vi "Power Output Retrieve Key Array for  Config.vi"(8 "error in (no error)":errorcluster, 9 "Datasheets":T11, 10 "Key Array In":T12, 11 "Connection Refnum":T1) -> (0 "error out":errorcluster, 2 "Power Output Test Parameters":T2={"Stimulus"={"Frequency Type"=enum."Band Edges", "Frequency Ranges"=[], "TX 1 Frequency (MHz)"={"Min"=0.0, "Max"=0.0}, "TX 2 Frequency (MHz)"={"Min"=0.0, "Max"=0.0}, "RX Frequency (MHz)"={"Min"=0.0, "Max"=0.0}, "Pad Model Number"="", "Pad Serial Number"="", "Pad Values"=[]}, "Measurement"={"DUT Port"=enum."Port 1", "Direction"=0, "Frequency Step Size"=0}, "Display"={"Frequency"={"Min"=-1.0, "Max"=-1.0}, "Power"={"Min"=-1, "Max"=-1}}, "Limit"={"Min Power (dBm)"=44.0}, "Calibration"={"Calibrated?"=FALSE}} {"Measurement"."Frequency Step Size" items=["0.2", "0.4", "1.0", "2.0", "4.0"]; "Measurement"."Direction" items=["Reverse", "Forward", "Auxiliary"]}, 3 "Connection Refnum":T1)   [LabVIEW 2011]
uses:
  Addons/internet/utils/keyedarr.llb/Keyed Array.ctl
  Test Datasheets.ctl
  TypeDefs/Power Output Test Parameters.ctl
  TypeDefs/Power Output Stimulus Parameters.ctl
  TypeDefs/Power Output Measurement Parameters.ctl
  SI.LIB/PIM.LIB/HW IO/DUTport.ctl
  SI.LIB/PIM.LIB/HW IO/MeasMode.ctl
  SI.LIB/PIM.LIB/HW IO/PIM Sweep Step Size.ctl
  TypeDefs/Power Output Display Parameters.ctl
  TypeDefs/Power Output Limit Parameters.ctl
  TypeDefs/Power Output Calibration State.ctl
  SI.LIB/ODBC/SQL Controls/Connection Refnum.ctl
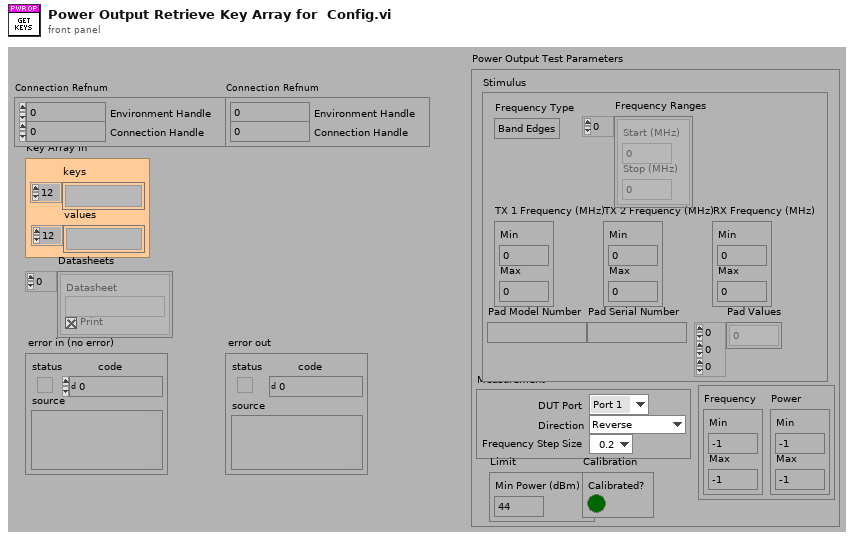
[diagram p1: front panel]
types:
  T1 = typedef "Connection Refnum.ctl" = cluster{"Environment Handle":i32, "Connection Handle":i32}
  T2 = typedef "Power Output Test Parameters.ctl" = cluster{"Stimulus":T3, "Measurement":T4, "Display":T8, "Limit":T9, "Calibration":T10}
  T3 = typedef "Power Output Stimulus Parameters.ctl" = cluster{"Frequency Type":enum16{"Band Edges", "Custom"}, "Frequency Ranges":cluster{"Start (MHz)":dbl, "Stop (MHz)":dbl}[], "TX 1 Frequency (MHz)":cluster{"Min":dbl, "Max":dbl}, "TX 2 Frequency (MHz)":cluster{"Min":dbl, "Max":dbl}, "RX Frequency (MHz)":cluster{"Min":dbl, "Max":dbl}, "Pad Model Number":string, "Pad Serial Number":string, "Pad Values":dbl[][][]}
  T4 = typedef "Power Output Measurement Parameters.ctl" = cluster{"DUT Port":T5, "Direction":T6, "Frequency Step Size":T7}
  T5 = typedef "DUTport.ctl" = enum16{"Port 1", "Port 2"}
  T6 = typedef "MeasMode.ctl" = u16
  T7 = typedef "PIM Sweep Step Size.ctl" = u16
  T8 = typedef "Power Output Display Parameters.ctl" = cluster{"Frequency":cluster{"Min":dbl, "Max":dbl}, "Power":cluster{"Min":i32, "Max":i32}}
  T9 = typedef "Power Output Limit Parameters.ctl" = cluster{"Min Power (dBm)":dbl}
  T10 = typedef "Power Output Calibration State.ctl" = cluster{"Calibrated?":bool}
  T11 = typedef "Test Datasheets.ctl" = cluster{"Datasheet":string, "Print":bool}[]
  T12 = typedef "Keyed Array.ctl" = cluster{"keys":string[], "values":string[]}
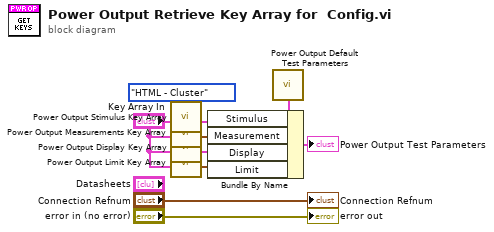
[diagram p0: block diagram]
diagram:
  w3 = enum16{"Cluster - HTML", "HTML - Cluster"}."HTML - Cluster" ("Conversion")
  n1 = call "Power Output Stimulus Key Array.vi"("Conversion"=w3, "Stimulus Key Array In"="Key Array In") -> ("Stimulus Cluster Out"=w7:T3)  [unwired: 5 in, 1 out]
  n2 = call "Power Output Measurements Key Array.vi"("Conversion"=w3, "Measurements Key Array In"="Key Array In") -> ("Measurements Cluster Out"=w6:T4)  [unwired: 5 in, 1 out]
  n3 = call "Power Output Display Key Array.vi"("Conversion"=w3, "Display Key Array In"="Key Array In") -> ("Display Cluster Out"=w5:T8)  [unwired: 5 in, 1 out]
  n4 = call "Power Output Limit Key Array.vi"("Conversion"=w3, "Limits Key Array In"="Key Array In") -> ("Limits Cluster Out"=w4:T9)  [unwired: 5 in, 1 out]
  n5 = call "Power Output Default Test Parameters.vi"() -> ("Default Power Output Test Parameters"=w8:T2)
  n6 = Bundle By Name(cluster=w8, "Stimulus"=w7, "Measurement"=w6, "Display"=w5, "Limit"=w4) -> (→"Power Output Test Parameters":T2)
  "error out" <- "error in (no error)"
  "Connection Refnum" <- "Connection Refnum"
